vi "Get Cluster Element by Name__ogtk_TS.vi"(8 "error in (no error)":errorcluster, 9 "Element Name":string, 10 "Cluster":variant) -> (0 "error out":errorcluster, 1 "found?":bool, 2 "VElement":variant)   [LabVIEW 2011]
doc: "Returns the element in the cluster by its name."
panel:
  out "array":string[](array[string])
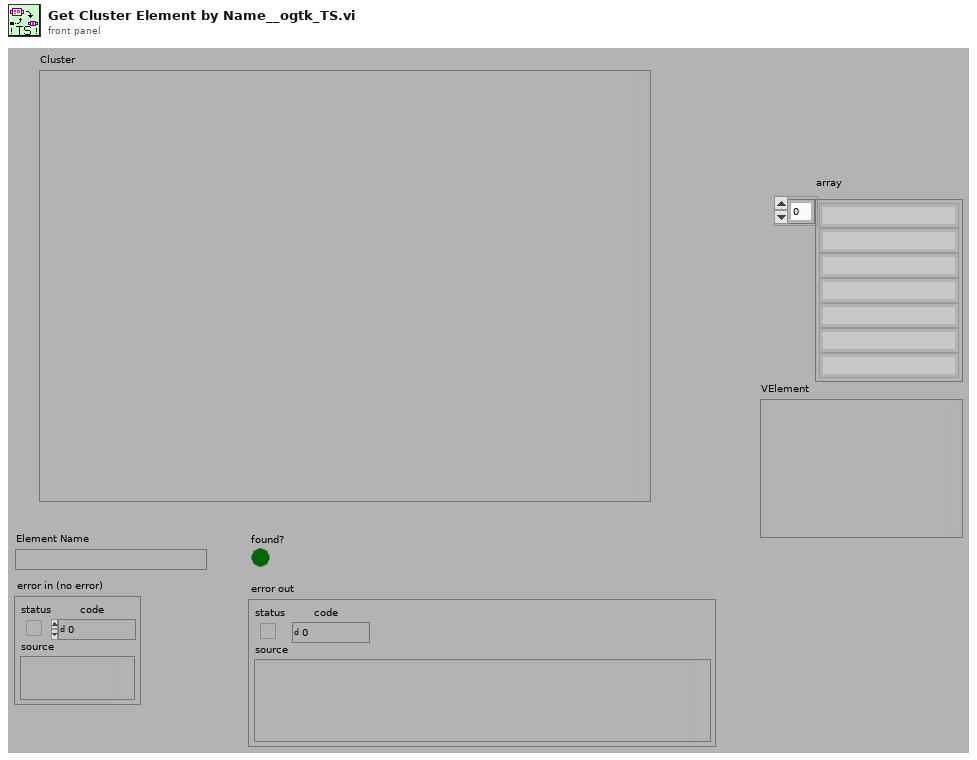
[diagram p1: front panel]
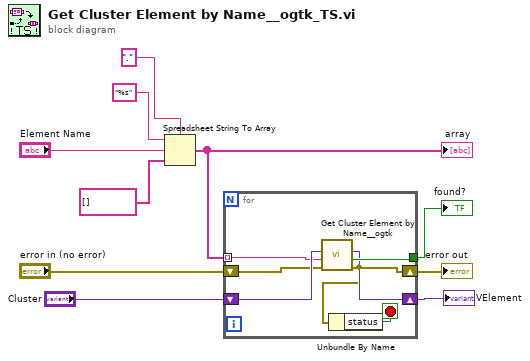
[diagram p0: block diagram]
diagram:
  n1 = Spreadsheet String To Array(delimiter (Tab)=".", format string="%s", spreadsheet string="Element Name", array type (2D Dbl)=string[] []) -> (array=w6:string[])
  "array" <- w6
  n2 = for {
    shift-right: [w14] -> w4
    shift-left: "Cluster" -> [w17]
    tunnel: w6 -> [w11] mode=indexing
    tunnel: [w16] -> w5
    shift-right: [w13] -> w3
    shift-left: "error in (no error)" -> [w15]
    stop <- w12 stop-if-true
    n3 = call "Get Cluster Element by Name__ogtk.vi"("error in (no error)"=w15, "Element Name"=w11, "Cluster"=w17) -> ("error out"=w13:errorcluster, "found?"=w16:bool, "VElement"=w14:variant)  [unwired: 6 in]
    n4 = Unbundle By Name(w13) -> ("status"=w12:bool)
  }
  "error out" <- w3
  "VElement" <- w4
  "found?" <- w5
